vi "test Get TagDistance By Tag ID.vi"(8 "error in (no error)":errorcluster, 11 "TestCase in":refnum<class "AnchorTests.lvclass">) -> (0 "error out":errorcluster, 3 "TestCase out":refnum<class "AnchorTests.lvclass">)   [LabVIEW 2014, in "AnchorTests.lvclass"]
uses:
  AnchorTests.lvclass
  SPLAT/Tag.lvclass
  <vilib>/addons/_JKI Toolkits/VI Tester/TestCase.llb/TestCase.lvclass
  SPLAT/Anchor/Anchor.lvclass
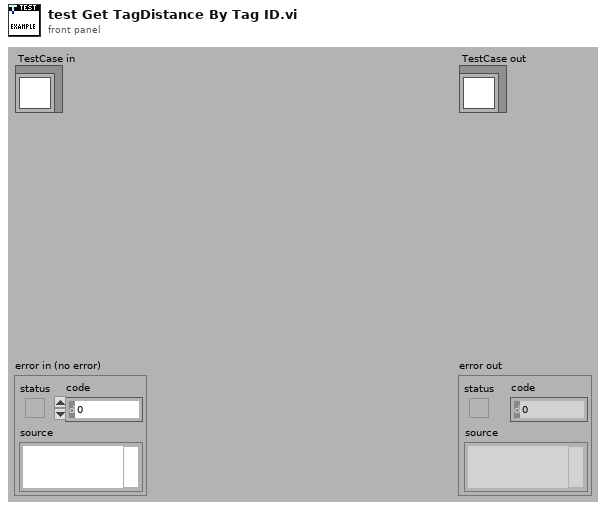
[diagram p1: front panel]
types:
  T1 = cluster{"Tag.lvclass":refnum<class "Tag.lvclass">, "Distance":dbl}[]
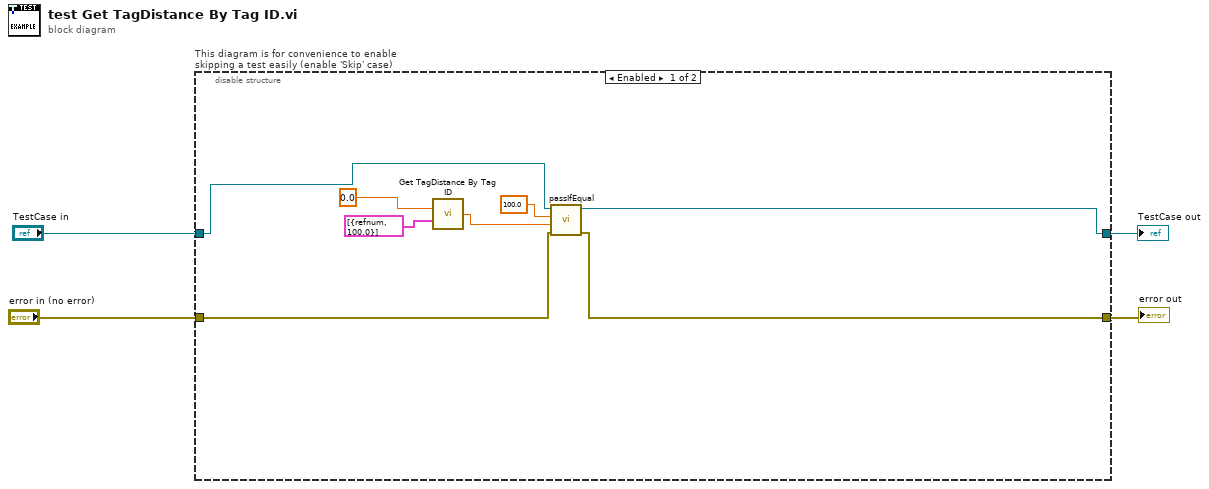
[diagram p0: block diagram]
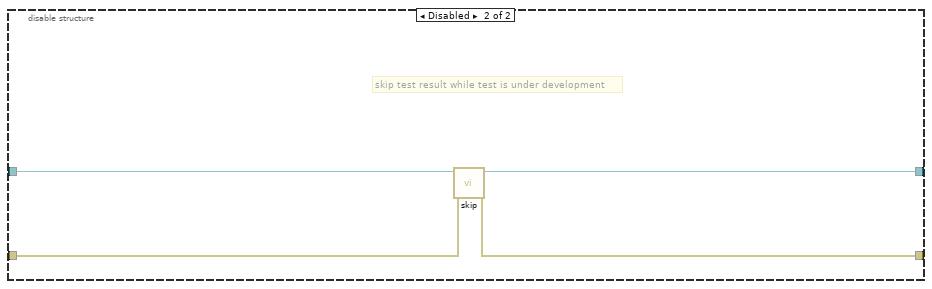
[diagram p2: hidden frame]
diagram:
  n1 = disable-structure "This diagram is for convenience to enable skipping a test easily (enable 'Skip' case)" shown="Enabled" {
    disable-tunnel: "TestCase in" -> [w9 w16]
    disable-tunnel: [w10 w14] -> w1
    disable-tunnel: [w7 w15] -> w3
    disable-tunnel: "error in (no error)" -> [w8 w13]
    frame Enabled {
      n2 = call "Get TagDistance By Tag ID.vi"("TagID"=0.0, "TagDistanceArray"=T1 [{"Tag.lvclass"=refnum, "Distance"=100.0}]) -> ("Distance"=w6:dbl)  [unwired: 13 in]
      n3 = call-dynamic "passIfEqual.vi"("error in (no error)"=w8, "y"=w6, "x"=100.0, "TestCase in"=w9) -> ("error out"=w7:errorcluster, "TestCase out"=w10:refnum<class "AnchorTests.lvclass">)  [unwired: 6 in]
    }
    frame Disabled {
      # "skip test result while test is under development"
      n4 = call <vilib>:"skip.vi"("error in (no error)"=w13, "TestCase in"=w16) -> ("error out"=w15:errorcluster, "TestCase out"=w14:refnum<class "AnchorTests.lvclass">)  [unwired: 8 in]
    }
  }
  "error out" <- w3
  "TestCase out" <- w1
